vi "Set DC Motors.vi"(4 "DC motor 1 error (0)":i32, 6 "DC motor 0 error (0)":i32, 8 "error in (no error)":errorcluster, 9 "DC motor 1 (right)":refnum<class "DC Motor Controller.lvclass">, 10 "DC motor 0 (left)":refnum<class "DC Motor Controller.lvclass">, 11 "NI_Robotics_Starter Kit Host in":refnum<class "NI_Robotics_Starter Kit Host.lvclass">) -> (0 "error out":errorcluster, 3 "NI_Robotics_Starter Kit Host out":refnum<class "NI_Robotics_Starter Kit Host.lvclass">)   [LabVIEW 2017, in "NI_Robotics_Starter Kit Host.lvclass"]
uses:
  <vilib>/robotics/Starter Kit/Host Interface/NI_Robotics_Starter Kit Host.lvclass
  <instrlib>/DC Motor Controller/HAIOL/DC Motor Controller.lvclass
  <vilib>/robotics/Starter Kit/Host Interface/NI_Robotics_Starter Kit Host.lvclass/NI_Robotics_Starter Kit Host.ctl
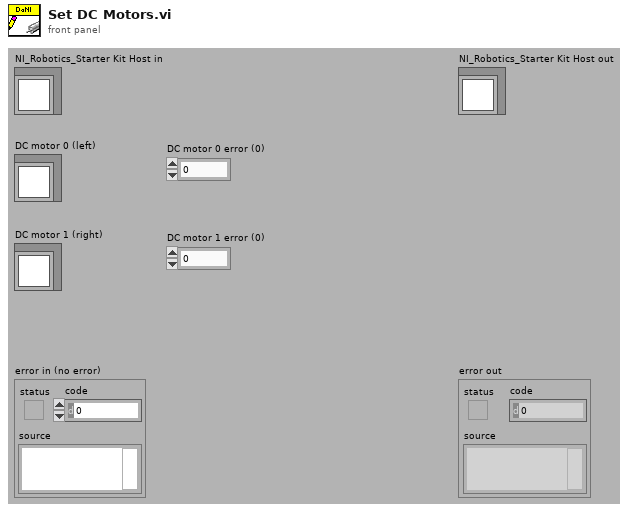
[diagram p1: front panel]
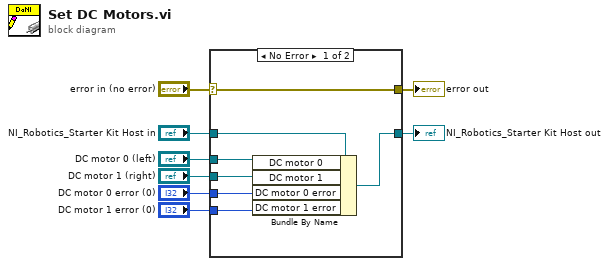
[diagram p0: block diagram]
diagram:
  n1 = case shown="No Error" "error in (no error)" {
    selector: "error in (no error)" -> [w15 w16]
    tunnel: [w15 w16] -> w7
    tunnel: [w13 w17] -> w5
    tunnel: "NI_Robotics_Starter Kit Host in" -> [w14 w17]
    tunnel: "DC motor 0 (left)" -> [w12 _]
    tunnel: "DC motor 1 (right)" -> [w11 _]
    tunnel: "DC motor 0 error (0)" -> [w10 _]
    tunnel: "DC motor 1 error (0)" -> [w9 _]
    frame No Error {
      n2 = Bundle By Name(cluster=w14, "DC motor 0"=w12, "DC motor 1"=w11, "DC motor 0 error"=w10, "DC motor 1 error"=w9) -> (w13:refnum<class "NI_Robotics_Starter Kit Host.lvclass">)
    }
    frame Error {
    }
  }
  "error out" <- w7
  "NI_Robotics_Starter Kit Host out" <- w5
